vi "All Neighbors.vi"(7 "Goal":T2, 11 "Position":T2) -> (2 "Froms":T1[](array[typedef]), 3 "All Neighbors":T2[](array[typedef]), 5 "Dirs":T1[](array[typedef]))   [LabVIEW 2020]
uses:
  Position.ctl
  Dir.ctl
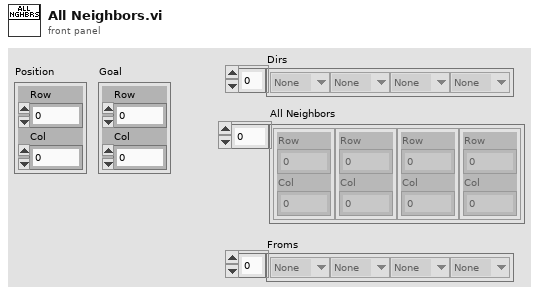
[diagram p1: front panel]
types:
  T1 = typedef "Dir.ctl" = enum16{"None", "Up", "Left", "Down", "Right"}
  T2 = typedef "Position.ctl" = cluster{"Row":i32, "Col":i32}
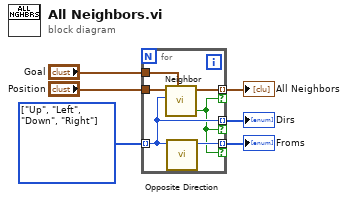
[diagram p0: block diagram]
diagram:
  w6 = T1[] [enum."Up", enum."Left", enum."Down", enum."Right"] items=["None", "Up", "Left", "Down", "Right"]
  n1 = for {
    tunnel: w6 -> [w8] mode=indexing
    tunnel: "Position" -> [w12]
    tunnel: [w11] -> w3 mode=indexing if=w7
    tunnel: "Goal" -> [w10]
    tunnel: [w9] -> w2 mode=indexing if=w7
    tunnel: [w8] -> w1 mode=indexing if=w7
    n2 = call "Neighbor.vi"("Goal"=w10, "Dir"=w8, "Position"=w12) -> ("Neighbor"=w11:T2, "In Bounds"=w7:bool)  [unwired: 7 in]
    n3 = call "Opposite Direction.vi"("Dir"=w8) -> ("Opp"=w9:T1)  [unwired: 10 in]
  }
  "All Neighbors" <- w3
  "Froms" <- w2
  "Dirs" <- w1
